vi "Log File Name for Mode.vi"(9 "Mode":T1, 10 "base path":path) -> (1 "for input Mode":path, 2 "for Create New":path, 3 "for Append":path, 5 "for Overwrite":path)   [LabVIEW 2021, in "Logging.lvlib"]
doc: "Take 'base path' and format it for presentation in the UI."
uses:
  Logging.lvlib
  Logging Mode.ctl
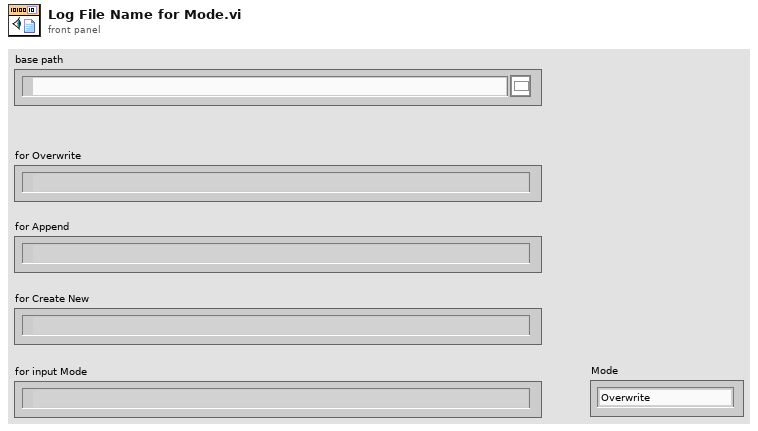
[diagram p1: front panel]
types:
  T1 = typedef "Logging.lvlib/Logging Mode.ctl" = enum16{"Overwrite", "Append", "Create New"}
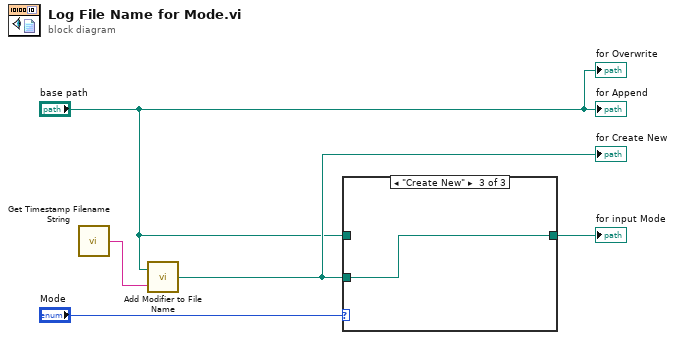
[diagram p0: block diagram]
diagram:
  n1 = call "Get Timestamp Filename String.vi"() -> ("time format string"=w5:string)
  n2 = call "Add Modifier to File Name.vi"("file name modifier"=w5, "base path"="base path") -> ("appended path"=w3:path)
  "for Create New" <- w3
  n3 = case shown="\"Create New\"" "Mode" {
    tunnel: w3 -> [_ _ w8]
    tunnel: "base path" -> [w6 w7 _]
    tunnel: [w6 w7 w8] -> w1
    frame "Overwrite" {
    }
    frame "Append" {
    }
    frame "Create New" {
    }
  }
  "for input Mode" <- w1
  "for Overwrite" <- "base path"
  "for Append" <- "base path"
